vi "View.vi"(8 "error in (no error)":errorcluster, 10 "Debugger":refnum<class "Debug Process.lvclass">, 11 "List View In":refnum<class "List Box View.lvclass">) -> (0 "error out":errorcluster, 3 "List View Out":refnum<class "List Box View.lvclass">)   [LabVIEW 2020, in "List Box View.lvclass"]
uses:
  List Box View.lvclass
  C:/Users/anton/Documents/GitHub/triarc-debugger/source/Debug View/Debug View.lvclass
  Process/Debug Process.lvclass
  Process/Debug Process.lvclass/Debug Process.ctl
  Debug View/Debug View.lvclass/Debug View.ctl
  List Box View.lvclass/List Box View.ctl
  Debug Data/Debug Data.lvclass
  List Box View Model_/List Box View Model.lvclass
  Debug View/Debug View.lvclass
panel:
  in  "Listbox":i32[](listbox)
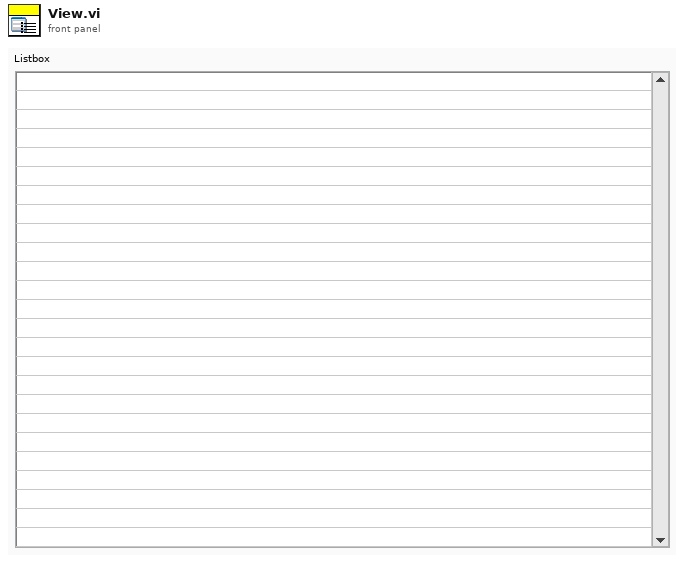
[diagram p1: front panel]
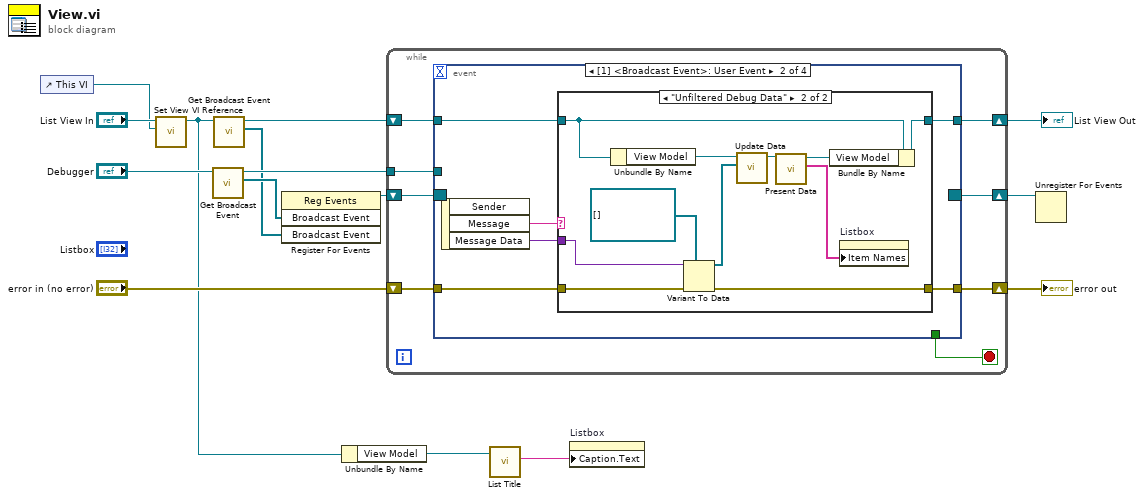
[diagram p0: block diagram]
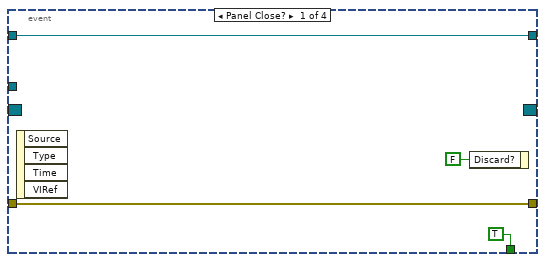
[diagram p2: hidden frame]
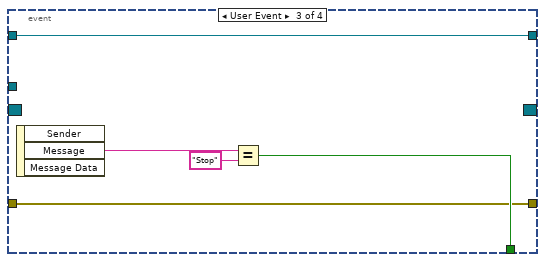
[diagram p4: hidden frame]
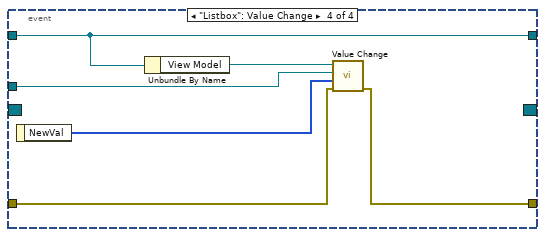
[diagram p5: hidden frame]
diagram:
  n1 = control-ref of="This VI"() -> (w1:refnum<vi>)
  n2 = call "Set View VI Reference.vi"("View VI ref"=w1, "Debug View in"="List View In") -> ("Debug View out"=w2:refnum<class "List Box View.lvclass">)  [unwired: 8 in, 1 out]
  n3 = call "Get Broadcast Event.vi"("Process in"="Debugger") -> ("Broadcast Event"=w6:refnum<user-event>[], "Process out"=w8:refnum<class "Debug Process.lvclass">)  [unwired: 8 in, 1 out]
  n4 = call "Get Broadcast Event.vi"("Debug View In"=w2) -> ("Broadcast Event"=w3:refnum<user-event>[], "Debug View Out"=w4:refnum<class "List Box View.lvclass">)  [unwired: 8 in, 1 out]
  n5 = register-events(w6, w3) -> (reference out=w7:refnum<event-registration>)  [unwired: 2 in, 1 out]
  n6 = Unbundle By Name(w2) -> ("View Model"=w11:refnum<class "List Box View Model.lvclass">)
  n7 = while {
    shift-right: [w22] -> w15
    shift-left: w4 -> [w23]
    shift-right: [w21] -> w14
    shift-left: "error in (no error)" -> [w20]
    shift-right: [w19] -> w12
    shift-left: w7 -> [w18]
    tunnel: w8 -> [w17]
    stop <- w16 stop-if-true
    n8 = event shown="[1] <Broadcast Event>: User Event" {
      selector: w18 -> [_ _ _ _]
      dyn-events: [_ _ _ _] -> w19
      timeout: _ -> [_ _ _ _]
      tunnel: w23 -> [w27 w29 w47 w57]
      tunnel: [w27 w28 w47 w57] -> w22
      tunnel: [w26 w32 w48 w53] -> w21
      tunnel: w20 -> [w26 w31 w48 w52]
      tunnel: w17 -> [_ _ _ w55]
      tunnel: [TRUE ("Discard?") _ w49 _] -> w16
      event Panel Close? {
        n9 = event-data() -> ()  [unwired: 1 in, 4 out]
        n10 = event-data("Discard?"=FALSE) -> ()  [unwired: 1 in, 1 out]
      }
      event User Event {
        n11 = event-data() -> ("Message"=w33:string, "Message Data"=w30:variant)  [unwired: 1 in, 1 out]
        n12 = case shown="\"Unfiltered Debug Data\"" w33 {
          tunnel: [w35 w45] -> w32
          tunnel: w31 -> [w35 w46]
          tunnel: w30 -> [_ w44]
          tunnel: w29 -> [w34 w42]
          tunnel: [w34 w39] -> w28
          frame Default {
          }
          frame "Unfiltered Debug Data" {
            n13 = Unbundle By Name(w42) -> ("View Model"=w41:refnum<class "List Box View Model.lvclass">)
            n14 = Variant To Data(error in=w46, type=refnum<class "Debug Data.lvclass">[] [] ("appended array"), Variant=w44) -> (data=w36:refnum<class "Debug Data.lvclass">[], error out=w45:errorcluster)
            n15 = call-dynamic "Update Data.vi"("Debug Data"=w36, "List Seen Processes View Model In"=w41) -> ("List Seen Processes View Model Out"=w37:refnum<class "List Box View Model.lvclass">)  [unwired: 8 in, 1 out]
            n16 = call "Present Data.vi"("List Seen Processes View Model In"=w37) -> ("Message List"=w40:string[], "List Seen Processes View Model Out"=w38:refnum<class "List Box View Model.lvclass">)  [unwired: 8 in, 1 out]
            n17 = Bundle By Name(cluster=w42, "View Model"=w38) -> (w39:refnum<class "List Box View.lvclass">)
            n18 = property on="Listbox" class="LstBox (strict)"("Item Names"=w40) -> ()  [unwired: 2 in, 2 out]
          }
        }
      }
      event User Event {
        n19 = event-data() -> ("Message"=w51:string)  [unwired: 1 in, 2 out]
        n20 = Equal?(x=w51, y="Stop") -> (x = y?=w49:bool)
      }
      event "Listbox": Value Change {
        n21 = event-data() -> ("NewVal"=w54:i32[])  [unwired: 1 in]
        n22 = Unbundle By Name(w57) -> ("View Model"=w56:refnum<class "List Box View Model.lvclass">)
        n23 = call-dynamic "Value Change.vi"("error in (no error)"=w52, "NewVal"=w54, "Debugger"=w55, "List Box View Model In"=w56) -> ("error out"=w53:errorcluster)  [unwired: 6 in, 1 out]
      }
    }
  }
  "error out" <- w14
  "List View Out" <- w15
  n24 = call-dynamic "List Title.vi"("List Box View Model in"=w11) -> ("Title"=w10:string)  [unwired: 8 in, 2 out]
  n25 = property on="Listbox" class="LstBox (strict)"("Caption.Text"=w10) -> ()  [unwired: 2 in, 2 out]
  n26 = Unregister For Events(event registration refnum=w12) -> ()  [unwired: 1 in, 1 out]
